vi "PackCommand.vi"(9 "data":string, 10 "unsigned byte array":u8[](array[numeric]), 11 "ISACommand":string) -> (3 "command":T1)   [LabVIEW 2017, in "ISA010_module.lvlib"]
uses:
  ISA010_module.lvlib
  ISA010/Command.ctl
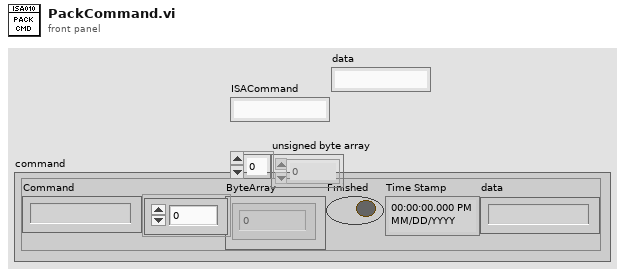
[diagram p1: front panel]
types:
  T1 = typedef "Command.ctl" = cluster{"Command":string, "ByteArray":u8[], "Finished":bool, "Time Stamp":timestamp, "data":string}
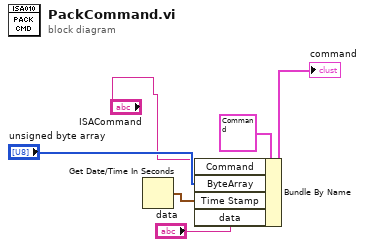
[diagram p0: block diagram]
diagram:
  n1 = Get Date/Time In Seconds() -> (seconds since 1Jan1904=w5:timestamp)
  n2 = Bundle By Name(cluster=T1 {"Command"="", "ByteArray"=[], "Finished"=FALSE, "Time Stamp"=timestamp(0 s since 1904-01-01), "data"=""} ("command"), "Command"="ISACommand", "ByteArray"="unsigned byte array", "Time Stamp"=w5, "data"="data") -> (→"command":T1)
